vi "核查数据断电保存 (子VI).vi"   [LabVIEW 2016, in "数据传输系统.lvlib"]
uses:
  <vilib>/Utility/config.llb/NI_LVConfig.lvlib
types:
  T1 = cluster{"setini":string, "sysini":string, "hechaini":string, "actualwrite":string, "actualread":string, "datasent":string, "反控命令信息队列":string, "反控与仪器交互":string}
  T2 = typedef "NI_LVConfig.lvlib/Config Data RefNum.ctl" = refnum<k1>
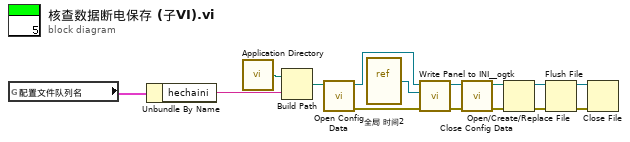
[diagram p0: block diagram]
diagram:
  n1 = global read "断电保存全局.vi" "配置文件队列名"() -> (w2:T1)
  n2 = Unbundle By Name(w2) -> ("hechaini"=w1:string)
  n3 = call <vilib>:"Application Directory.vi"() -> ("Application Directory"=w3:path)
  n4 = Build Path(base path=w3, name or relative path=w1) -> (appended path=w4:path)
  n5 = call <vilib>:"Open Config Data.vi"("configuration file path"=w4) -> ("error out"=w7:errorcluster, "refnum"=w15:T2)  [unwired: 8 in, 1 out]
  n6 = vi-ref "全局 时间2.vi"() -> (w5:refnum<vi>)
  n7 = call <userlib>:"Write Panel to INI__ogtk.vi"("error in (no error)"=w7, "VI ref"=w5, "refnum"=w15) -> ("error out"=w8:errorcluster, "refnum out"=w6:T2)  [unwired: 7 in]
  n8 = call <vilib>:"Close Config Data.vi"("error in (no error)"=w8, "refnum"=w6) -> ("error out"=w13:errorcluster, "file path"=w14:path)  [unwired: 8 in]
  n9 = Open/Create/Replace File(file path (use dialog)=w14, error in=w13) -> (refnum out=w10:refnum<file>, error out=w9:errorcluster)  [unwired: 4 in, 1 out]
  n10 = Flush File(refnum=w10, error in=w9) -> (refnum out=w11:refnum<file>, error out=w12:errorcluster)
  n11 = Close File(refnum=w11, error in=w12) -> ()  [unwired: 2 out]
